vi "全局 实时数据参数.vi"() -> ()   [LabVIEW 2016, in "数据传输系统-03.lvlib"]
panel:
  out "连接的字符串":string
  out "data":string[][](table)
  in  "参数":string
  in  "实时数据参数":string(combo)="水样测试"
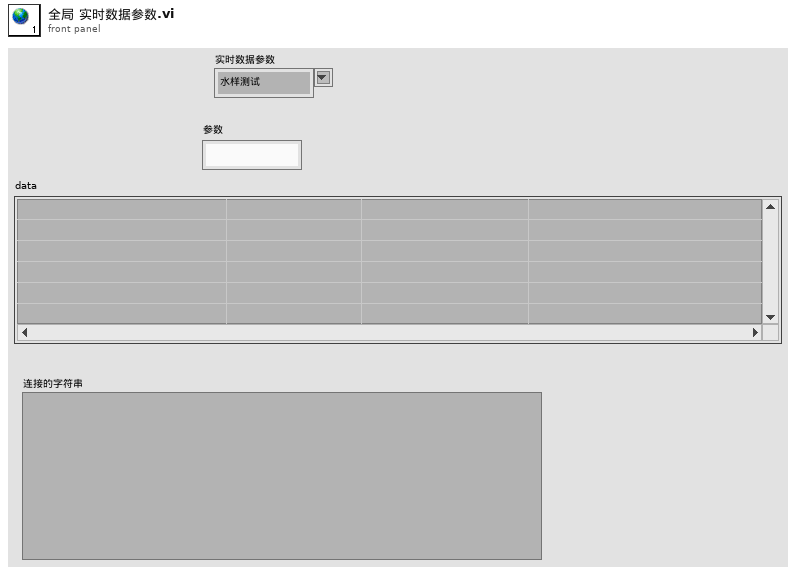
[diagram p1: front panel]
diagram:
